vi "Barrier Create Object.vi"(8 "error in (no error)":errorcluster, 11 "barrier pointer in":u64) -> (0 "error out":errorcluster, 3 "Barrier out":T1)   [LabVIEW 2013, in "POSIX Threads.lvlib" / "Barrier.lvclass"]
doc: "Creates a LabVIEW object used to encapsulate a pthread barrier object referenced by barrier pointer."
uses:
  Barrier.lvclass
  Controls/reference.ctl
  POSIX Thread Object/POSIX Thread Object.lvclass/POSIX Thread Object.ctl
  POSIX Thread Object/POSIX Thread Object.lvclass
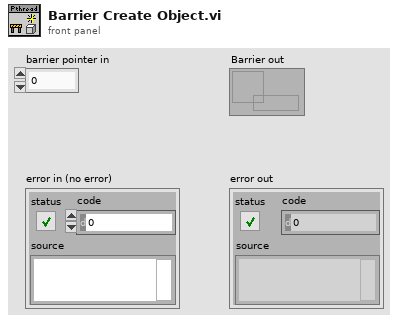
[diagram p1: front panel]
types:
  T1 = typedef "POSIX Threads.lvlib/Barrier.lvclass/reference.ctl" = refnum<data-value>
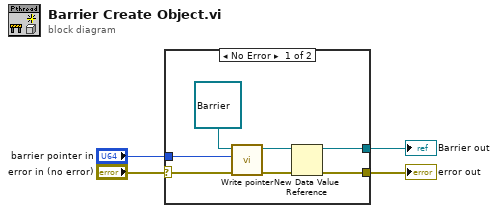
[diagram p0: block diagram]
diagram:
  n1 = case shown="No Error" "error in (no error)" {
    selector: "error in (no error)" -> [w8 w12]
    tunnel: "barrier pointer in" -> [w9 _]
    tunnel: [w7 w12] -> w2
    tunnel: [w6 _] -> w1
    frame No Error {
      n2 = call "Write pointer.vi"("error in (no error)"=w8, "pointer"=w9, "POSIX Thread Object in"=refnum<class "Barrier.lvclass"> refnum ("POSIX Threads.lvlib:Barrier")) -> ("error out"=w10:errorcluster, "POSIX Thread Object out"=w11:refnum<class "Barrier.lvclass">)  [unwired: 7 in]
      n3 = New Data Value Reference(data value=w11, error in=w10) -> (data value reference=w6:refnum<data-value>, error out=w7:errorcluster)
    }
    frame Error {
    }
  }
  "Barrier out" <- w1
  "error out" <- w2
